vi "Logging Message Loop.vi"(3 "UserMetaData":T1 {"Amplifier Model" items=["Select a Model", "AM 1700", "BMA 200"]}, 8 "error in (no error)":errorcluster, 10 "Data Queue":refnum<queue>, 11 "Message Queues":T2) -> (0 "error out":errorcluster)   [LabVIEW 2014, in "Logging.lvlib"]
doc: "The message loop subVI to handle messages pertaining to logging data."
uses:
  Logging.lvlib
  support/Message Queue/All Message Queues.ctl
  support/Message Queue/Message Cluster.ctl
  Logging Configuration.ctl
  Logging State.ctl
  support/Message Queue/Enqueue Message (Single).vi
  <vilib>/Utility/error.llb/Error Cluster From Error Code.vi
  <vilib>/ErrorRing/Error Ring.xnode
  support/Message Queue/Message Queue.lvlib
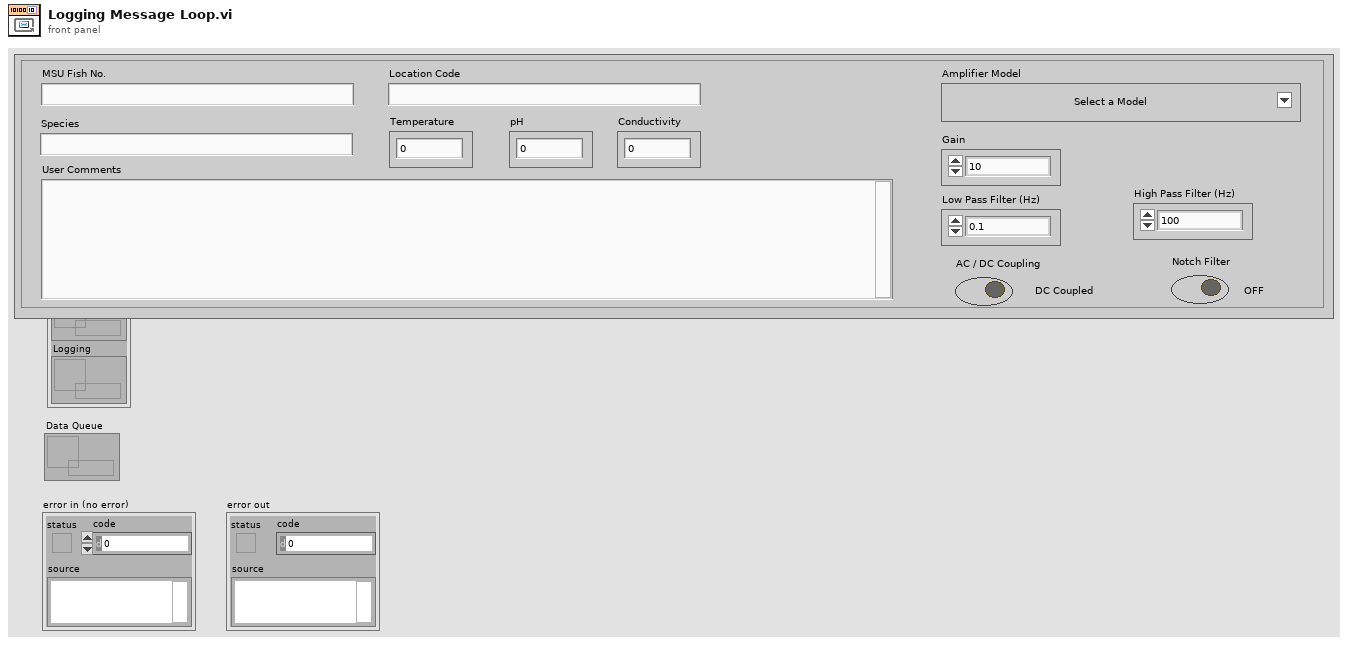
[diagram p1: front panel]
types:
  T1 = cluster{"MSU Fish No.":string, "Location Code":string, "Species":string, "Temperature":dbl, "pH":dbl, "Conductivity":dbl, "User Comments":string, "Amplifier Model":u16, "Gain":enum16{"10", "20", "50", "100", "200", "500", "1000", "2k", "5k", "10k", "20k", "50k"}, "Low Pass Filter (Hz)":enum16{"0.1", "1", "3", "10", "30", "100", "300"}, "High Pass Filter (Hz)":enum16{"100", "500", "1000", "3000", "5000", "10,000", "20,000", "30,000", "50,000"}, "AC / DC Coupling":bool, "Notch Filter":bool}
  T2 = typedef "Message Queue.lvlib/All Message Queues.ctl" = cluster{"UI":refnum<queue>, "Acquisition":refnum<queue>, "Logging":refnum<queue>}
  T3 = typedef "Logging.lvlib/Logging State.ctl" = cluster{"State":enum16{"Logging", "Not Logging", "Idle"}, "Samples to Save":u32, "Force Trigger":bool}
  T4 = typedef "Logging.lvlib/Logging Configuration.ctl" = cluster{"Log File Base Path":path, "TDMS File Reference":refnum<k34>, "Samples to Save":u32, "Trigger - Time":u32, "Trigger - Threshold":dbl, "Trigger - Channel":u32, "Enable Time Trigger":bool, "Enable Threshold Trigger":bool, "Always Log":bool}
  T5 = enum16{"open", "open or create", "create or replace", "create", "open (read-only)"}
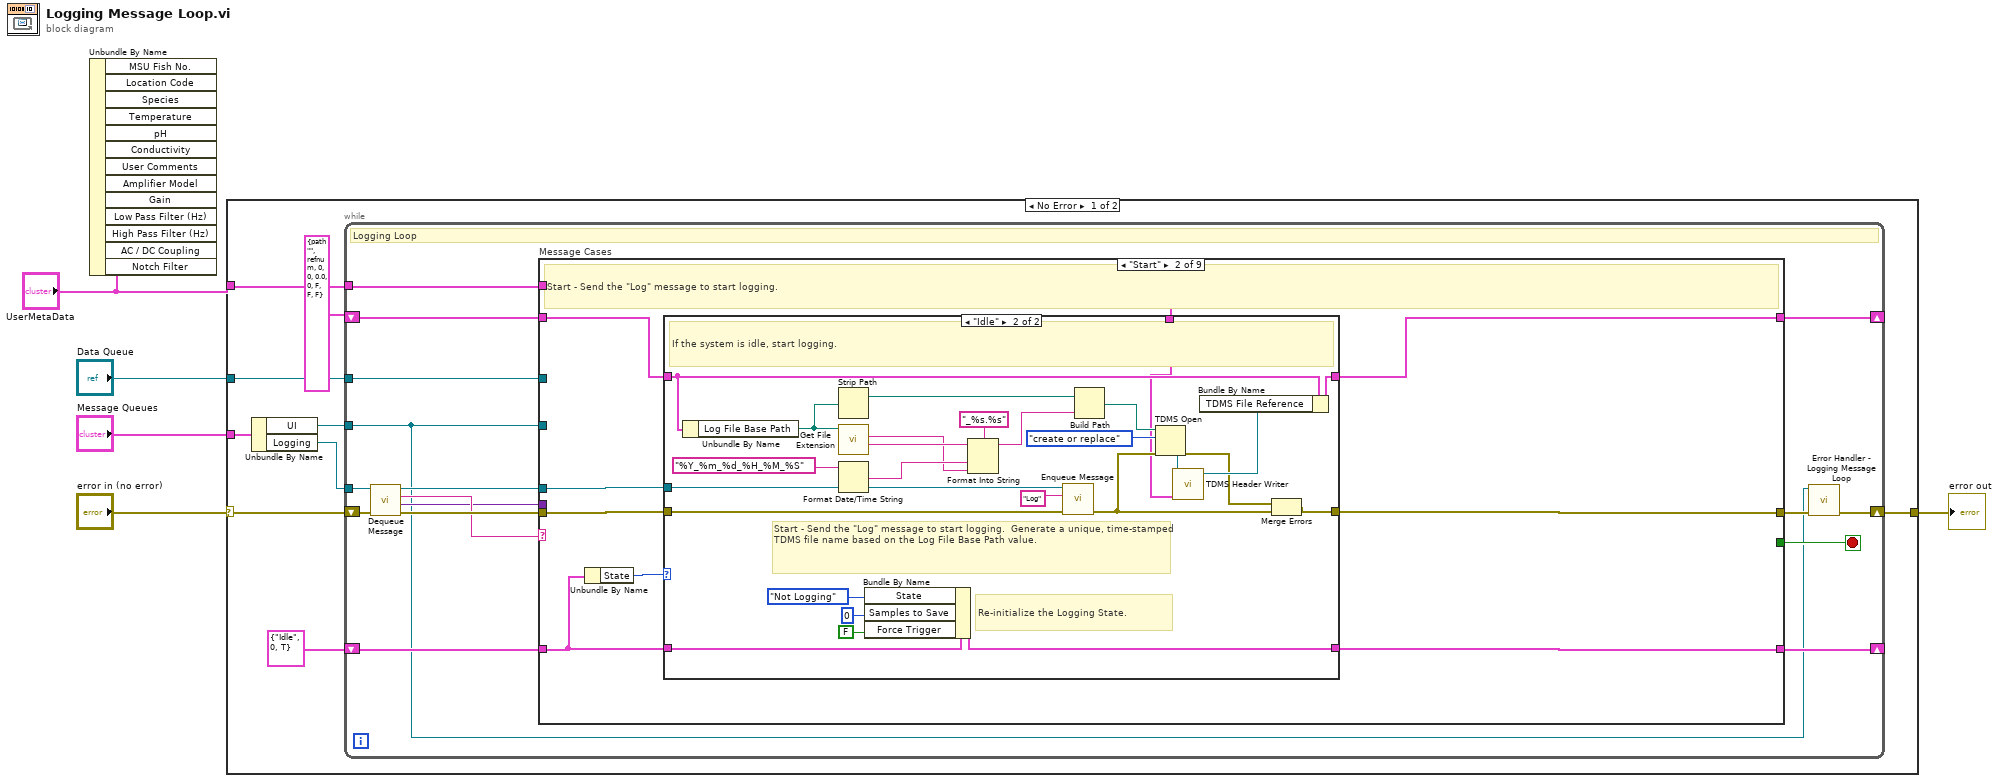
[diagram p0: block diagram]
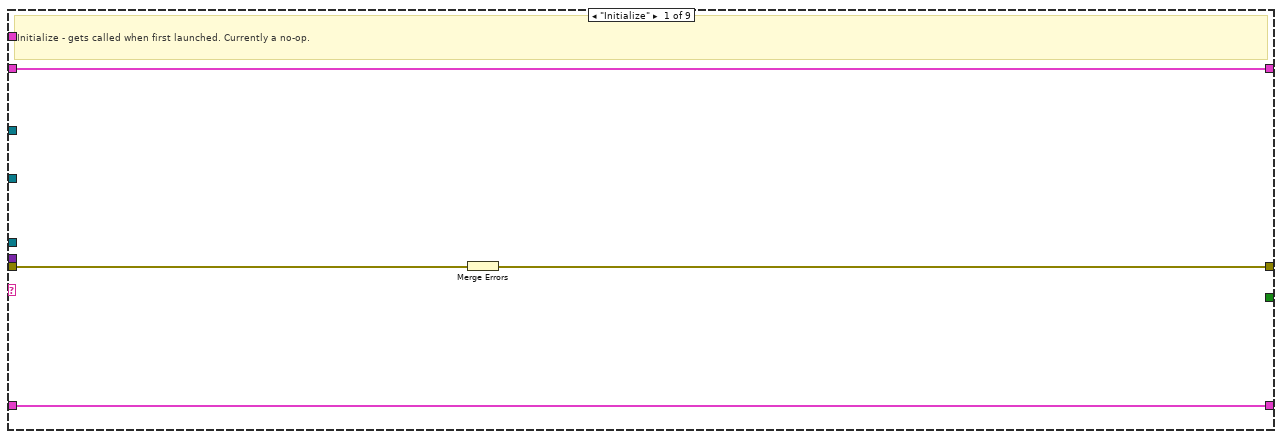
[diagram p2: hidden frame]
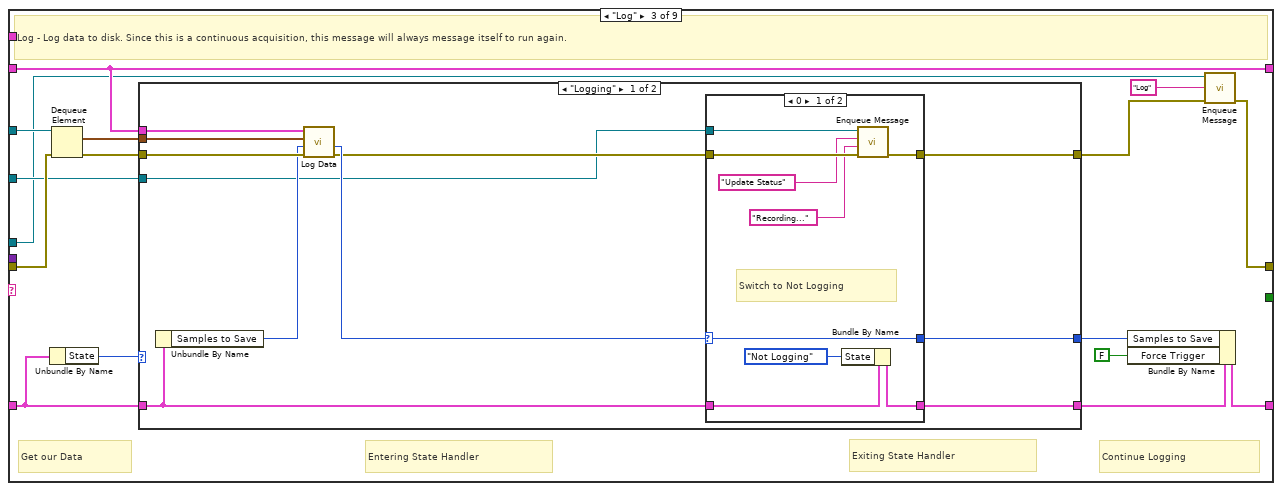
[diagram p4: hidden frame]
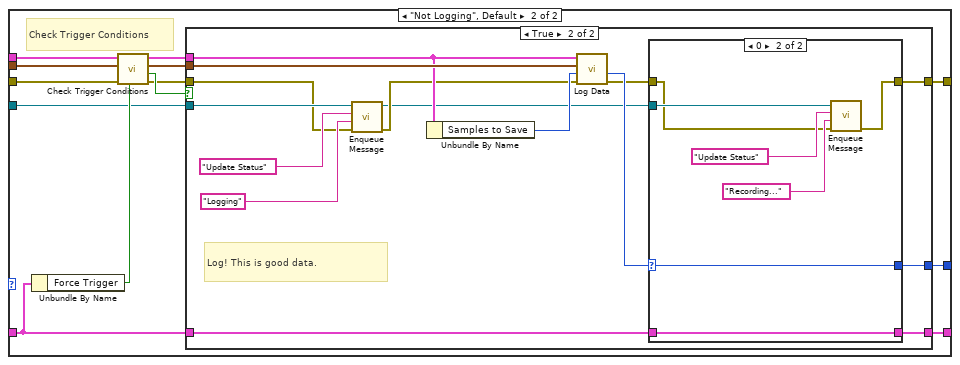
[diagram p6: hidden frame]
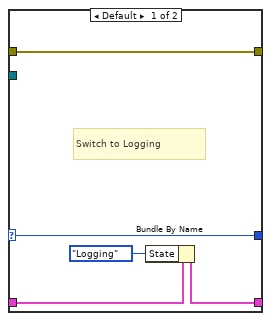
[diagram p8: hidden frame]
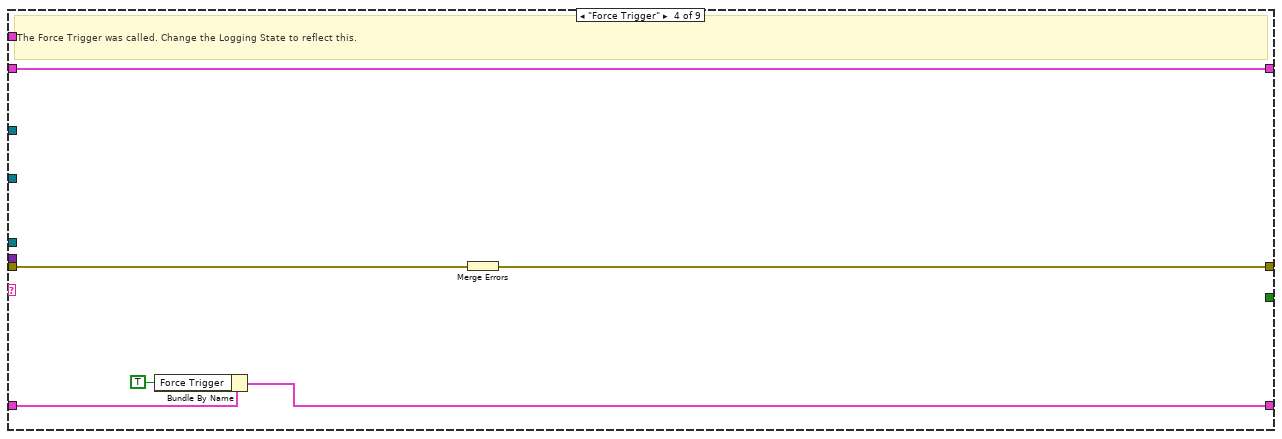
[diagram p9: hidden frame]
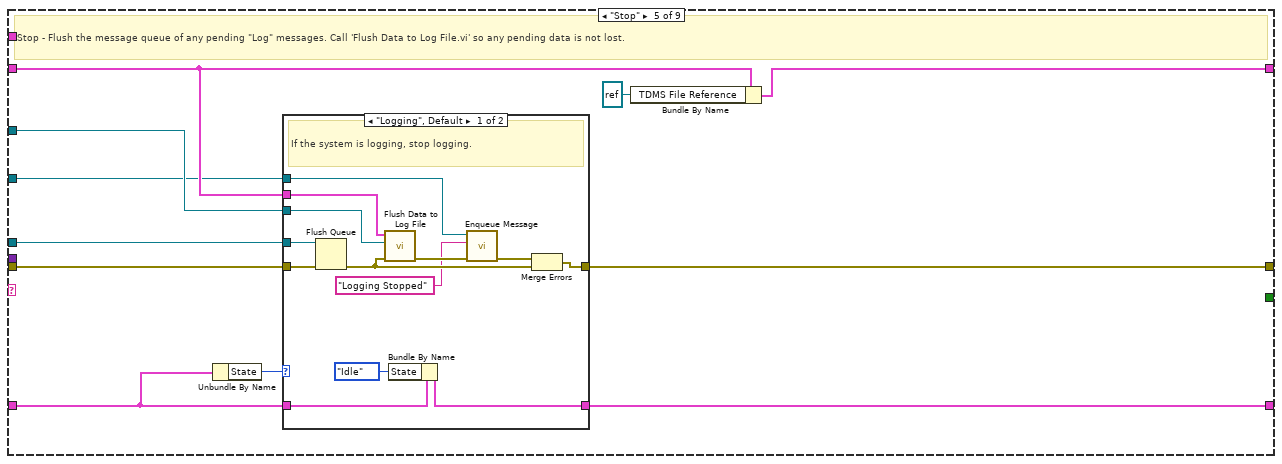
[diagram p10: hidden frame]
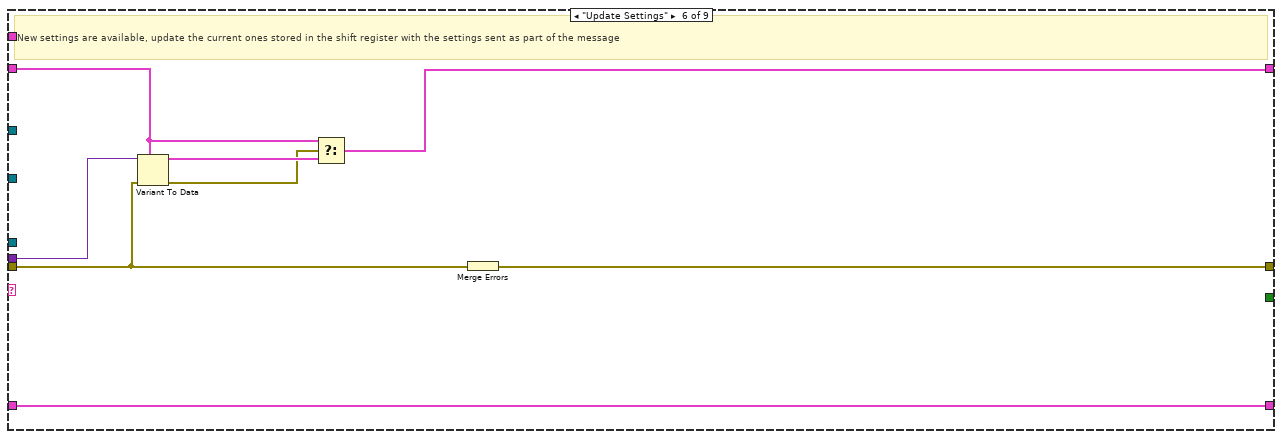
[diagram p12: hidden frame]
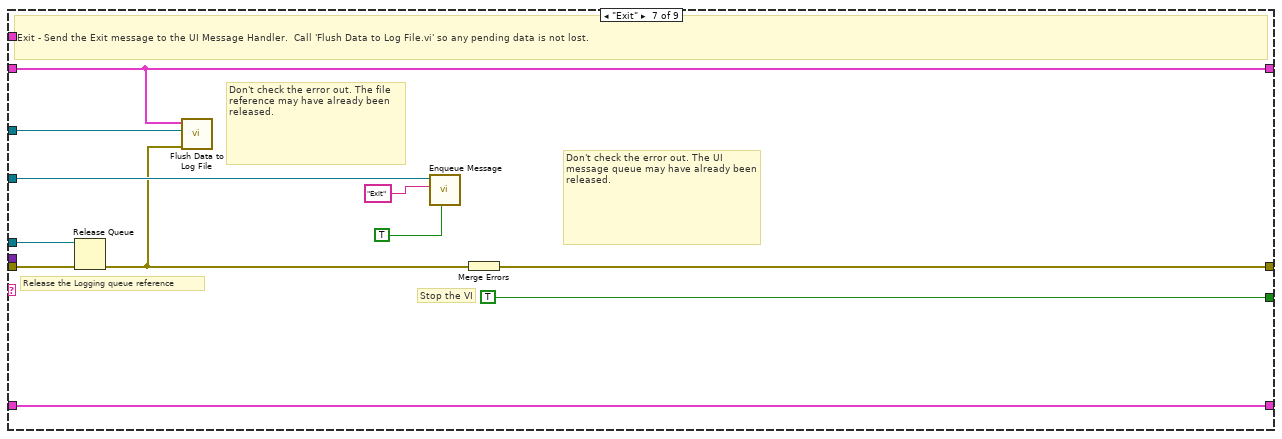
[diagram p13: hidden frame]
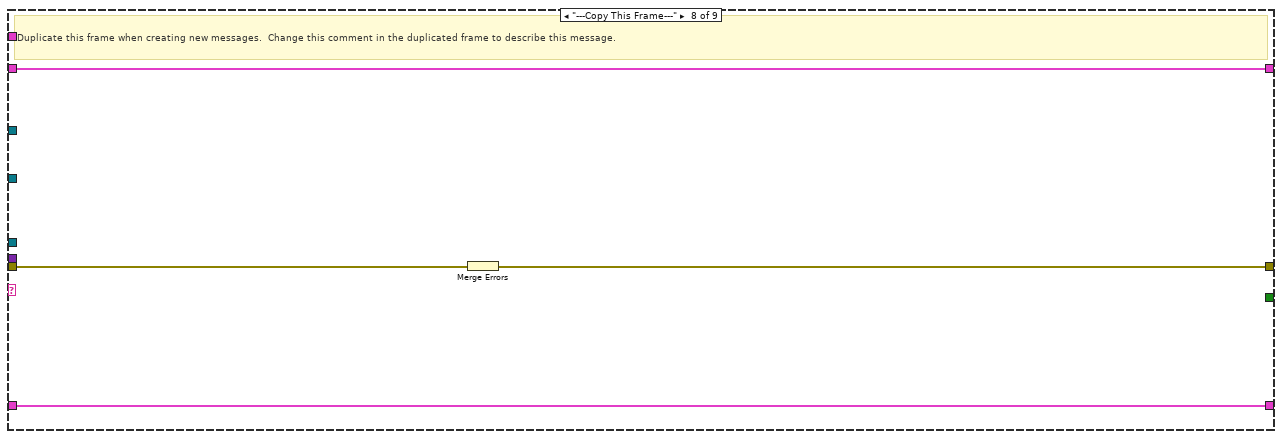
[diagram p14: hidden frame]
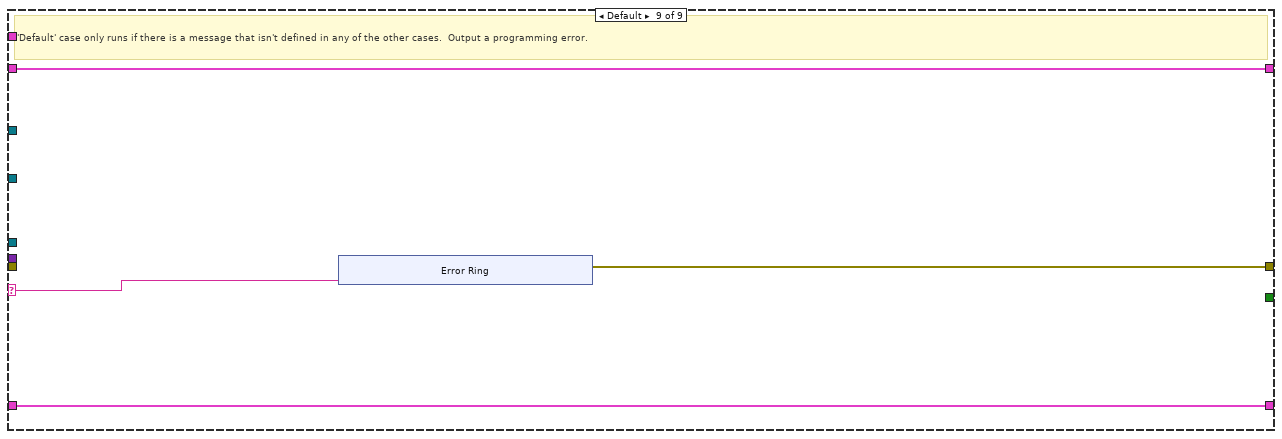
[diagram p15: hidden frame]
diagram:
  n1 = Unbundle By Name("UserMetaData") -> ()  [unwired: 13 out]
  n2 = case shown="No Error" "error in (no error)" {
    selector: "error in (no error)" -> [w10 w220]
    tunnel: "Message Queues" -> [w14 _]
    tunnel: [w12 w220] -> w4
    tunnel: "Data Queue" -> [w9 _]
    tunnel: "UserMetaData" -> [w6 _]
    frame No Error {
      n3 = Unbundle By Name(w14) -> ("UI"=w8:refnum<queue>, "Logging"=w13:refnum<queue>)
      n4 = while {
        tunnel: w13 -> [w22]
        shift-right: [w29] -> _
        shift-left: T4 {"Log File Base Path"=path "", "TDMS File Reference"=refnum, "Samples to Save"=0, "Trigger - Time"=0, "Trigger - Threshold"=0.0, "Trigger - Channel"=0, "Enable Time Trigger"=FALSE, "Enable Threshold Trigger"=FALSE, "Always Log"=FALSE} ("Logging Configuration") -> [w30]
        shift-right: [w17] -> w12
        shift-left: w10 -> [w27]
        tunnel: w8 -> [w16]
        tunnel: w9 -> [w21]
        shift-right: [w19] -> _
        shift-left: T3 {"State"=enum."Idle", "Samples to Save"=0, "Force Trigger"=TRUE} -> [w20]
        tunnel: w6 -> [w15]
        stop <- w28 stop-if-true
        # "Logging Loop"
        n5 = call "Dequeue Message.vi"("error in (no error)"=w27, "Message Queue"=w22) -> ("error out"=w26:errorcluster, "Message Data"=w24:variant, "Message"=w25:string, "dup Message Queue"=w23:refnum<queue>)  [unwired: 6 in]
        n6 = case "Message Cases" shown="\"Start\"" w25 {
          selector: w25 -> [_ _ _ _ _ _ _ _ w209]
          tunnel: w23 -> [_ w42 w76 _ w168 _ w198 _ _]
          tunnel: w26 -> [w32 w41 w86 w159 w169 w187 w201 w208 _]
          tunnel: [w34 w43 w88 w157 w170 w193 w203 w206 w210] -> w18
          tunnel: w30 -> [w33 w40 w81 w158 w165 w191 w197 w207 w212]
          tunnel: [w33 w39 w81 w158 w167 w188 w197 w207 w212] -> w29
          tunnel: [_ _ _ _ _ _ TRUE _ _] -> w28
          tunnel: w24 -> [_ _ _ _ _ w192 _ _ _]
          tunnel: w16 -> [_ _ w80 _ w163 _ w202 _ _]
          tunnel: w21 -> [_ _ w77 _ w164 _ w196 _ _]
          tunnel: w20 -> [w31 w37 w84 w156 w161 w186 w194 w205 w211]
          tunnel: [w31 w38 w79 w155 w160 w186 w194 w205 w211] -> w19
          tunnel: w15 -> [_ w35 _ _ _ _ _ _ _]
          frame "Initialize" {
            # "Initialize - gets called when first launched. Currently a no-op."
            n7 = Merge Errors(w32) -> (w34:errorcluster)
          }
          frame "Start" {
            # "Start - Send the \"Log\" message to start logging."
            n8 = Unbundle By Name(w37) -> ("State"=w36:enum16{"Logging", "Not Logging", "Idle"})
            n9 = case shown="\"Idle\"" w36 {
              tunnel: [w45 w72] -> w43
              tunnel: w42 -> [_ w71]
              tunnel: w41 -> [w45 w69]
              tunnel: w40 -> [w46 w60]
              tunnel: [w46 w58] -> w39
              tunnel: w37 -> [w44 w55]
              tunnel: [w44 w54] -> w38
              tunnel: w35 -> [_ w47]
              frame "Logging", Default {
                # "The system is already running. Ignore the \"Start\" message."
              }
              frame "Idle" {
                # "Re-initialize the Logging State."
                # "Start - Send the \"Log\" message to start logging.  Generate a unique, time-stamped TDMS file name based on the Log File Base Path value."
                # "If the system is idle, start logging."
                n10 = Unbundle By Name(w60) -> ("Log File Base Path"=w67:path)
                n11 = Strip Path(path=w67) -> (stripped path=w66:path)  [unwired: 1 out]
                n12 = call <vilib>:"Get File Extension.vi"("file"=w67) -> ("filename without extension"=w65:string, "lowercase file extension"=w62:string)  [unwired: 7 in, 2 out]
                n13 = Format Date/Time String(time format string (%c)="%Y_%m_%d_%H_%M_%S") -> (date/time string=w63:string)  [unwired: 2 in]
                n14 = Bundle By Name(cluster=w55, "State"=enum16{"Logging", "Not Logging"}."Not Logging", "Samples to Save"=u32 0 ("Reads to Save"), "Force Trigger"=FALSE) -> (w54:T3)
                n15 = Format Into String(format string="_%s.%s", initial string=w65, w63, w62) -> (resulting string=w61:string)  [unwired: 1 in, 1 out]
                n16 = call-poly "Enqueue Message.vi"("error in (no error)"=w69, "Message"="Log", "Message Queue"=w71) -> ("error out"=w56:errorcluster)  [unwired: 7 in, 1 out]
                n17 = Build Path(base path=w66, name or relative path=w61) -> (appended path=w59:path)
                n18 = TDMS Open(8:w56, 10:T5."create or replace" ("operation (0:open)"), 11:w59) -> (0:w48:errorcluster, 3:w50:refnum<k34>)  [unwired: 4 in]
                n19 = call "TDMS Header Writer.vi"("UserMetaData"=w47, "tdms file"=w50) -> ("tdms file out"=w49:refnum<k34>)  [unwired: 7 in, 2 out]
                n20 = Bundle By Name(cluster=w60, "TDMS File Reference"=w49) -> (w58:T4)
                n21 = Merge Errors(w48, w56) -> (w72:errorcluster)
              }
            }
          }
          frame "Log" {
            # "Exiting State Handler"
            # "Continue Logging"
            # "Entering State Handler"
            # "Get our Data"
            # "Log - Log data to disk. Since this is a continuous acquisition, this message will always message itself to run again."
            n22 = Unbundle By Name(w84) -> ("State"=w85:enum16{"Logging", "Not Logging", "Idle"})
            n23 = Dequeue Element(queue=w77, error in (no error)=w86) -> (element=w83:waveform(dbl)[], error out=w82:errorcluster)  [unwired: 1 in, 2 out]
            n24 = case shown="\"Logging\"" w85 {
              tunnel: [w93 w116] -> w75
              tunnel: w84 -> [w94 w114]
              tunnel: w83 -> [w98 w123]
              tunnel: w82 -> [w97 w122]
              tunnel: w81 -> [w99 w124]
              tunnel: w80 -> [w89 w113]
              tunnel: [w90 w115] -> w73
              tunnel: [w92 w112] -> w74
              frame "Logging" {
                n25 = Unbundle By Name(w94) -> ("Samples to Save"=w96:u32)
                n26 = call "Log Data.vi"("error in (no error)"=w97, "Samples to Save In"=w96, "Data"=w98, "Logging Configuration"=w99) -> ("error out"=w91:errorcluster, "Samples to Save Out"=w95:u32)  [unwired: 6 in]
                n27 = case shown="0" w95 {
                  selector: w95 -> [w105 w111]
                  tunnel: w91 -> [w103 w110]
                  tunnel: [w104 w110] -> w90
                  tunnel: w94 -> [w107 w109]
                  tunnel: [w106 w109] -> w93
                  tunnel: [w105 w111] -> w92
                  tunnel: w89 -> [w100 _]
                  frame 0 {
                    # "Switch to Not Logging"
                    n28 = Bundle By Name(cluster=w107, "State"=enum16{"Logging", "Not Logging"}."Not Logging") -> (w106:T3)
                    n29 = call-poly "Enqueue Message.vi"("error in (no error)"=w103, "Message Data"="Recording..." ("Waiting for trigger"), "Message"="Update Status", "Message Queue"=w100) -> ("error out"=w104:errorcluster)  [unwired: 6 in, 1 out]
                  }
                  frame Default {
                    # "Continue in our same State."
                  }
                }
              }
              frame "Not Logging", Default {
                # "Check Trigger Conditions"
                n30 = Unbundle By Name(w114) -> ("Force Trigger"=w121:bool)
                n31 = call "Check Trigger Conditions.vi"("Force Trigger?"=w121, "error in (no error)"=w122, "Waveform Data In"=w123, "Logging Configuration In"=w124) -> ("error out"=w119:errorcluster, "Trigger Conditions Met?"=w120:bool, "Waveform Data Out (copy)"=w118:waveform(dbl)[], "Logging Configuration Out"=w117:T4)  [unwired: 4 in]
                n32 = case shown="True" w120 {
                  tunnel: w119 -> [w125 w135]
                  tunnel: w118 -> [_ w141]
                  tunnel: w117 -> [_ w140]
                  tunnel: w114 -> [w126 w131]
                  tunnel: [w126 w130] -> w116
                  tunnel: [w125 w128] -> w115
                  tunnel: w113 -> [_ w139]
                  tunnel: [_ w132] -> w112
                  frame False {
                  }
                  frame True {
                    # "Log! This is good data."
                    n33 = call-poly "Enqueue Message.vi"("error in (no error)"=w135, "Message Data"="Logging" ("Logging"), "Message"="Update Status", "Message Queue"=w139) -> ("error out"=w134:errorcluster, "dup Message Queue"=w127:refnum<queue>)  [unwired: 6 in]
                    n34 = Unbundle By Name(w140) -> ("Samples to Save"=w136:u32)
                    n35 = call "Log Data.vi"("error in (no error)"=w134, "Samples to Save In"=w136, "Data"=w141, "Logging Configuration"=w140) -> ("error out"=w129:errorcluster, "Samples to Save Out"=w133:u32)  [unwired: 6 in]
                    n36 = case shown="0" w133 {
                      selector: w133 -> [w146 w153]
                      tunnel: [w146 w153] -> w132
                      tunnel: [w143 w152] -> w130
                      tunnel: w131 -> [w144 w152]
                      tunnel: w129 -> [w142 w148]
                      tunnel: [w142 w147] -> w128
                      tunnel: w127 -> [_ w151]
                      frame Default {
                        # "Switch to Logging"
                        n37 = Bundle By Name(cluster=w144, "State"=enum16{"Logging", "Not Logging"}."Logging") -> (w143:T3)
                      }
                      frame 0 {
                        n38 = call-poly "Enqueue Message.vi"("error in (no error)"=w148, "Message Data"="Recording..." ("Waiting for trigger"), "Message"="Update Status", "Message Queue"=w151) -> ("error out"=w147:errorcluster)  [unwired: 6 in, 1 out]
                      }
                    }
                  }
                }
              }
            }
            n39 = Bundle By Name(cluster=w75, "Samples to Save"=w74, "Force Trigger"=FALSE) -> (w79:T3)
            n40 = call-poly "Enqueue Message.vi"("error in (no error)"=w73, "Message"="Log", "Message Queue"=w76) -> ("error out"=w88:errorcluster)  [unwired: 7 in, 1 out]
          }
          frame "Force Trigger" {
            # "The Force Trigger was called. Change the Logging State to reflect this."
            n41 = Bundle By Name(cluster=w156, "Force Trigger"=TRUE) -> (w155:T3)
            n42 = Merge Errors(w159) -> (w157:errorcluster)
          }
          frame "Stop" {
            # "Stop - Flush the message queue of any pending \"Log\" messages. Call 'Flush Data to Log File.vi' so any pending data is not lost."
            n43 = Unbundle By Name(w161) -> ("State"=w162:enum16{"Logging", "Not Logging", "Idle"})
            n44 = case shown="\"Logging\", Default" w162 {
              tunnel: [w183 w185] -> w170
              tunnel: w169 -> [w182 w185]
              tunnel: w168 -> [w181 _]
              tunnel: w165 -> [w180 _]
              tunnel: w164 -> [w179 _]
              tunnel: w163 -> [w175 _]
              tunnel: w161 -> [w173 w184]
              tunnel: [w172 w184] -> w160
              frame "Logging", Default {
                # "If the system is logging, stop logging."
                n45 = Flush Queue(queue=w181, error in (no error)=w182) -> (error out=w178:errorcluster)  [unwired: 2 out]
                n46 = call "Flush Data to Log File.vi"("error in (no error)"=w178, "Data Queue"=w179, "Logging Configuration"=w180) -> ("error out"=w177:errorcluster)  [unwired: 8 in]
                n47 = Bundle By Name(cluster=w173, "State"=enum16{"Logging", "Not Logging", "Idle"}."Idle") -> (w172:T3)
                n48 = call-poly "Enqueue Message.vi"("error in (no error)"=w177, "Message"="Logging Stopped", "Message Queue"=w175) -> ("error out"=w176:errorcluster)  [unwired: 7 in, 1 out]
                n49 = Merge Errors(w176, w178) -> (w183:errorcluster)
              }
              frame "Idle" {
                # "The system is already idle. Ignore the \"Stop\" message."
              }
            }
            n50 = Bundle By Name(cluster=w165, "TDMS File Reference"=refnum<k34> refnum ("tdms file out")) -> (w167:T4)
          }
          frame "Update Settings" {
            # "New settings are available, update the current ones stored in the shift register with the settings sent as part of the message"
            n51 = Variant To Data(error in=w187, type=w191, Variant=w192) -> (data=w190:T4, error out=w189:errorcluster)
            n52 = Select(t=w191, s=w189, f=w190) -> (s? t:f=w188:T4)
            n53 = Merge Errors(w187) -> (w193:errorcluster)
          }
          frame "Exit" {
            # "Don't check the error out. The file reference may have already been released."
            # "Release the Logging queue reference"
            # "Don't check the error out. The UI message queue may have already been released."
            # "Stop the VI"
            # "Exit - Send the Exit message to the UI Message Handler.  Call 'Flush Data to Log File.vi' so any pending data is not lost."
            n54 = Release Queue(queue=w198, error in (no error)=w201) -> (error out=w195:errorcluster)  [unwired: 1 in, 2 out]
            n55 = call "Flush Data to Log File.vi"("error in (no error)"=w195, "Data Queue"=w196, "Logging Configuration"=w197) -> ()  [unwired: 8 in, 1 out]
            n56 = call-poly "Enqueue Message.vi"("Priority Message? (F)"=TRUE, "Message"="Exit", "Message Queue"=w202) -> ()  [unwired: 7 in, 2 out]
            n57 = Merge Errors(w195) -> (w203:errorcluster)
          }
          frame "---Copy This Frame---" {
            # "Duplicate this frame when creating new messages.  Change this comment in the duplicated frame to describe this message."
            n58 = Merge Errors(w208) -> (w206:errorcluster)
          }
          frame Default {
            # "'Default' case only runs if there is a message that isn't defined in any of the other cases.  Output a programming error."
            n59 = xnode "Error Ring"("parameter 0"=w209) -> ("error out"=w210:errorcluster)
          }
        }
        n60 = call "Error Handler - Logging Message Loop.vi"("error in (no error)"=w18, "Message Queue"=w16) -> ("dup error in"=w17:errorcluster)  [unwired: 8 in, 1 out]
      }
    }
    frame Error {
    }
  }
  "error out" <- w4
